vi "Acquire.vi"(8 "error in (no error)":errorcluster, 9 "Data Queue":refnum<queue>, 10 "Data Notifier":refnum<notifier>, 11 "Hardware Resources in":T1) -> (0 "error out":errorcluster, 3 "Hardware Resources out":T1)   [LabVIEW 2016, in "Acquisition.lvlib"]
doc: "Perform the acquisition. Replace the contents of this diagram with calls to acquisition hardware."
uses:
  Acquisition.lvlib
  Hardware Configuration.ctl
  <vilib>/DAQmx/read.llb/DAQmx Read (Analog 1D Wfm NChan NSamp).vi
  <vilib>/DAQmx/miscellaneous.llb/DAQmx Fill In Error Info.vi
  <resource>/objmgr/daqmx.rc
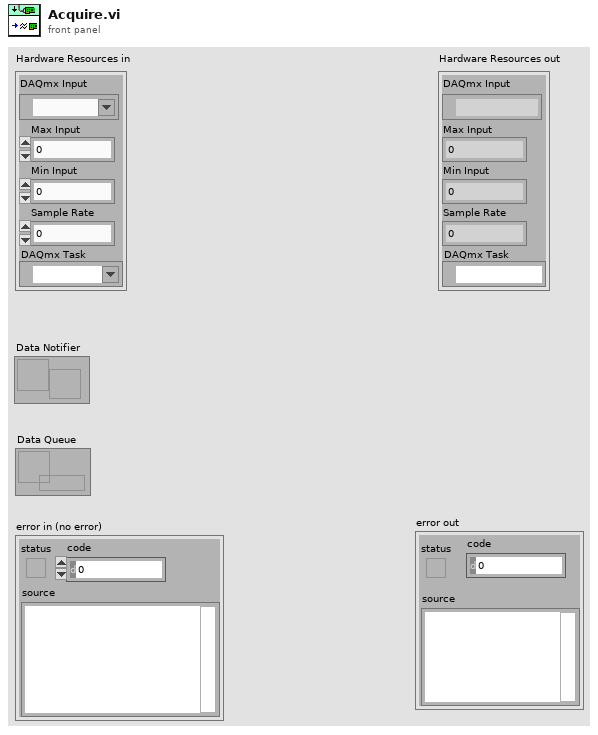
[diagram p1: front panel]
types:
  T1 = typedef "Acquisition.lvlib/Hardware Configuration.ctl" = cluster{"DAQmx Input":tag, "Max Input":dbl, "Min Input":dbl, "Sample Rate":dbl, "DAQmx Task":refnum<k21>}
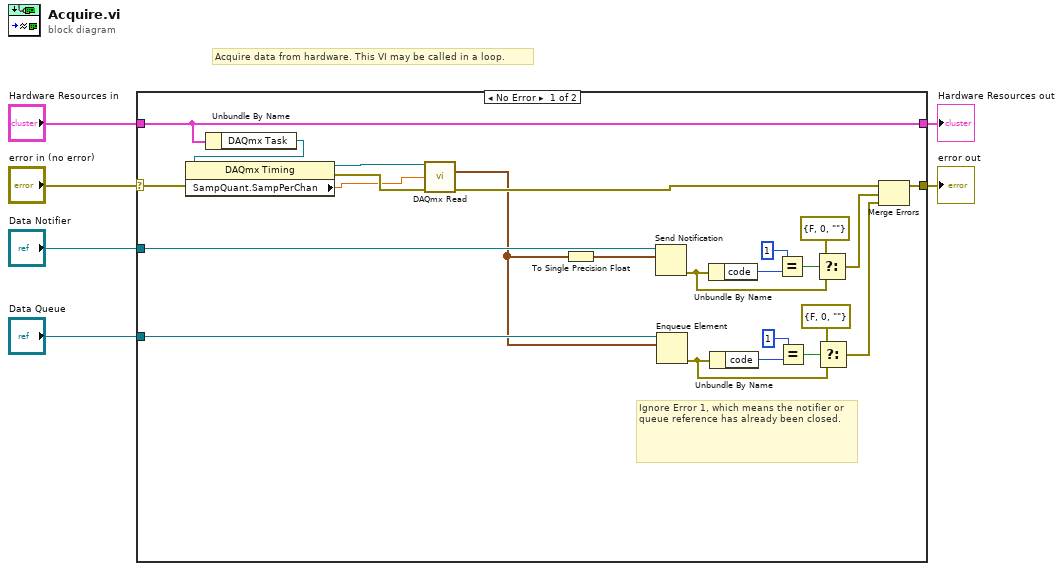
[diagram p0: block diagram]
diagram:
  # "Acquire data from hardware. This VI may be called in a loop."
  n1 = case shown="No Error" "error in (no error)" {
    selector: "error in (no error)" -> [w10 w31]
    tunnel: [w30 w31] -> w5
    tunnel: "Hardware Resources in" -> [w15 w32]
    tunnel: [w15 w32] -> w3
    tunnel: "Data Notifier" -> [w29 _]
    tunnel: "Data Queue" -> [w16 _]
    frame No Error {
      # "Ignore Error 1, which means the notifier or queue reference has already been closed."
      n2 = Unbundle By Name(w15) -> ("DAQmx Task"=w12:refnum<k21>)
      n3 = property class="DAQmx Timing"(reference=w12, error in=w10) -> (reference out=w11:refnum<k21>, error out=w9:errorcluster, "SampQuant.SampPerChan"=w8:dbl)
      n4 = call-poly <vilib>:"DAQmx Read.vi"("task/channels in"=w11, "number of samples per channel"=w8, "error in"=w9) -> ("data"=w13:waveform(dbl)[], "error out"=w14:errorcluster)  [unwired: 10 in, 1 out]
      n5 = To Single Precision Float(number=w13) -> (single precision float=w7:waveform(sgl)[])
      n6 = Send Notification(notification=w7, notifier=w29) -> (error out=w25:errorcluster)  [unwired: 1 in, 1 out]
      n7 = Enqueue Element(queue=w16, element=w13) -> (error out=w21:errorcluster)  [unwired: 2 in, 2 out]
      n8 = Unbundle By Name(w25) -> ("code"=w28:i32)
      n9 = Unbundle By Name(w21) -> ("code"=w18:i32)
      n10 = Equal?(x=1, y=w28) -> (x = y?=w26:bool)
      n11 = Equal?(x=1, y=w18) -> (x = y?=w20:bool)
      n12 = Select(t=errorcluster {"status"=FALSE, "code"=0, "source"=""} ("error constant"), s=w26, f=w25) -> (s? t:f=w24:errorcluster)
      n13 = Select(t=errorcluster {"status"=FALSE, "code"=0, "source"=""} ("error constant"), s=w20, f=w21) -> (s? t:f=w17:errorcluster)
      n14 = Merge Errors(w14, w24, w17) -> (w30:errorcluster)
    }
    frame Error {
    }
  }
  "Hardware Resources out" <- w3
  "error out" <- w5
